vi "TDMSAdv readData.vi"(6 "stringSplit? (T)":bool=TRUE, 7 "readEvent":T1, 8 "error in (no error)":errorcluster, 10 "timeStamp":string, 11 "TDMSAdv in":refnum<class "TDMSAdv.lvclass">) -> (0 "error out":errorcluster, 2 "outputArr":string[][](array[string]), 3 "TDMSAdv out":refnum<class "TDMSAdv.lvclass">, 5 "getListTag":string[](array[string])=["TimeStamp", "SampleType", "mzRange"])   [LabVIEW 2018, in "TDMSAdv.lvclass"]
uses:
  TDMSAdv.lvclass
  FM/ctl/_PC_Pub_FM fileReadFuncEnum.ctl
  TDMSAdv.lvclass/TDMSAdv.ctl
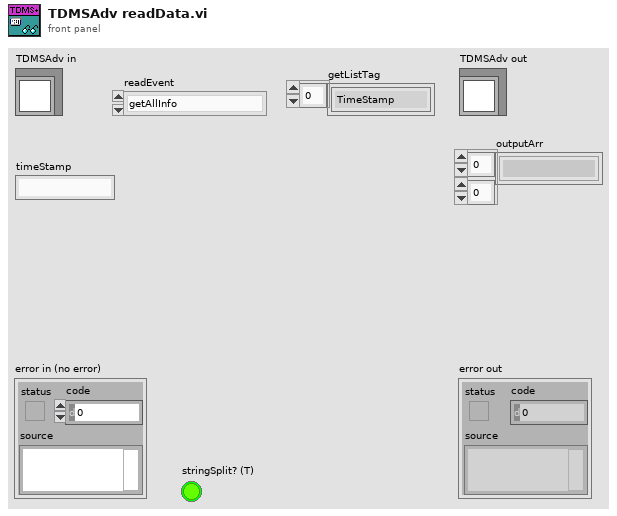
[diagram p1: front panel]
types:
  T1 = typedef "_PC_Pub_FM fileReadFuncEnum.ctl" = enum16{"getAllInfo", "getChromatogram", "getDataItems", "getTimeStamp", "getIdxData", "getIonization", "getRemark", "getAttrFormat"}
  T2 = enum16{"open", "open or create", "create or replace", "create", "open (read-only)"}
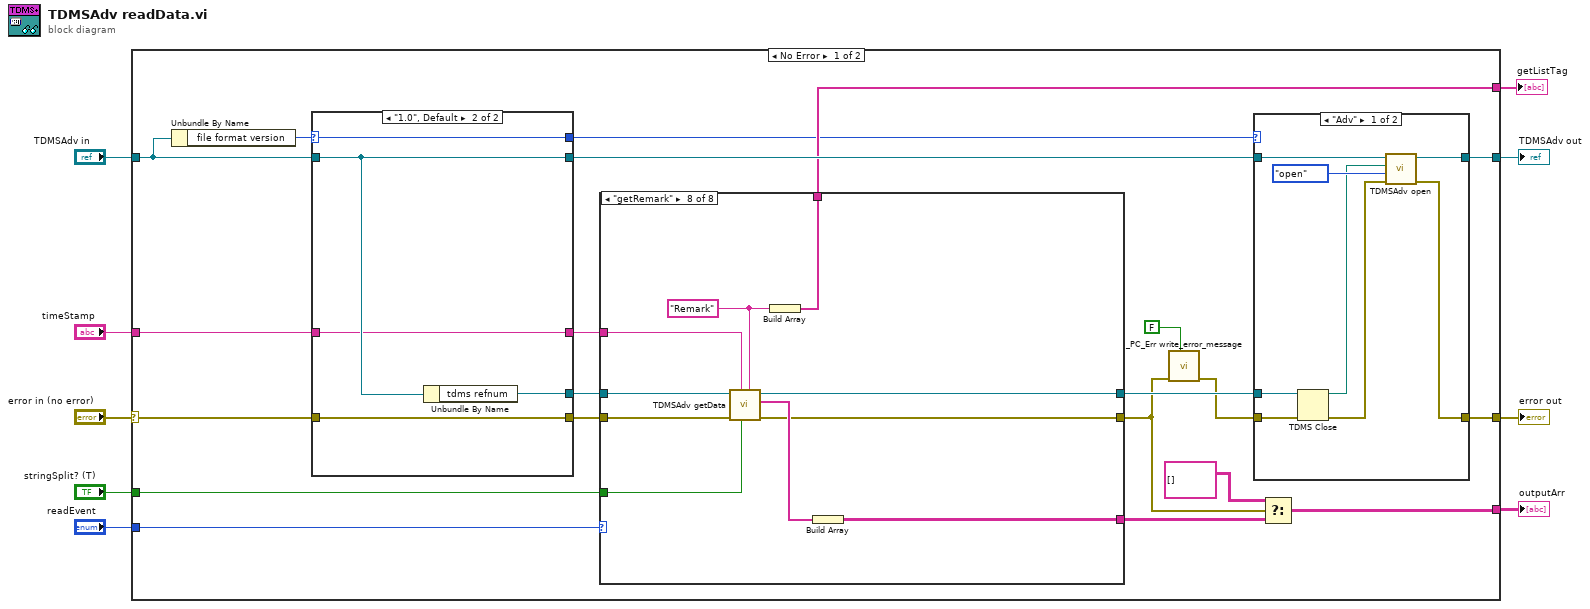
[diagram p0: block diagram]
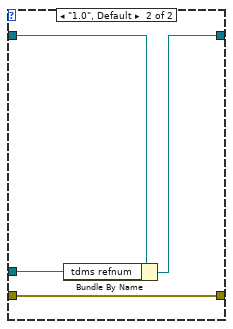
[diagram p2: hidden frame]
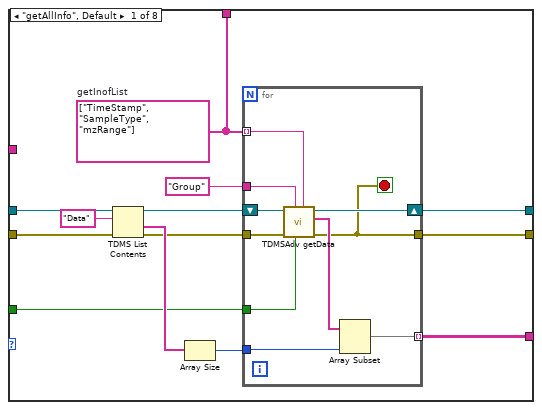
[diagram p3: hidden frame]
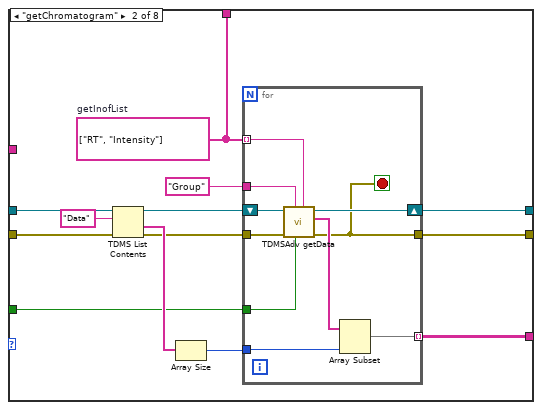
[diagram p4: hidden frame]
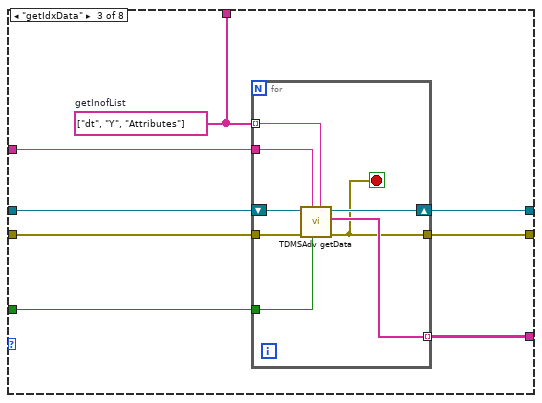
[diagram p5: hidden frame]
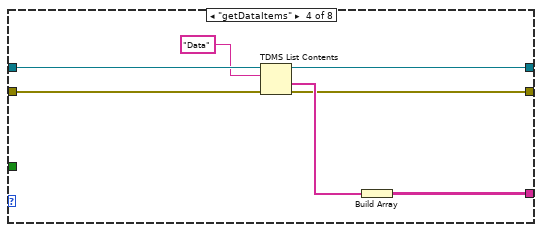
[diagram p6: hidden frame]
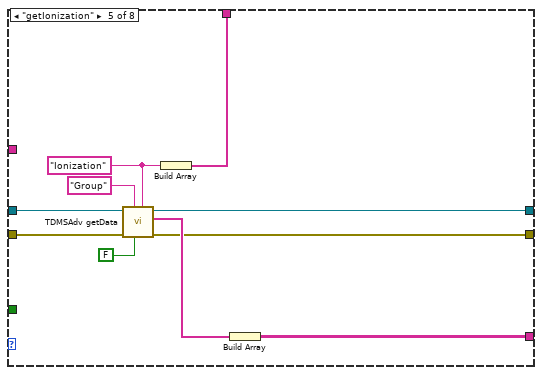
[diagram p7: hidden frame]
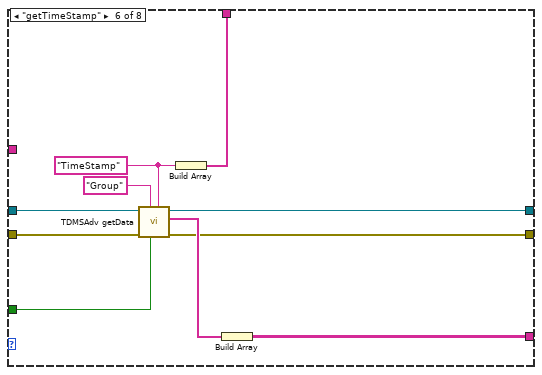
[diagram p8: hidden frame]
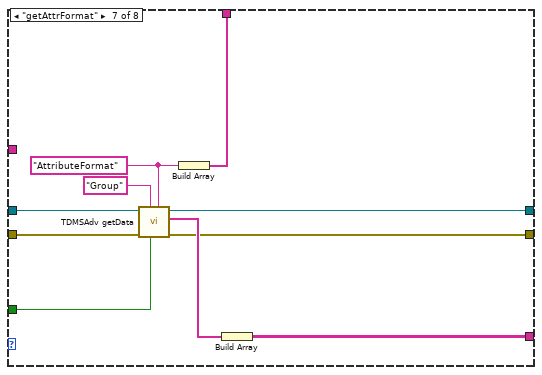
[diagram p9: hidden frame]
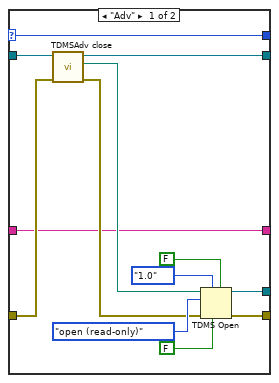
[diagram p10: hidden frame]
diagram:
  n1 = case shown="No Error" "error in (no error)" {
    selector: "error in (no error)" -> [w28 w170]
    tunnel: "TDMSAdv in" -> [w29 w171]
    tunnel: "timeStamp" -> [w20 _]
    tunnel: "readEvent" -> [w18 _]
    tunnel: "stringSplit? (T)" -> [w17 _]
    tunnel: [w15 _] -> w2
    tunnel: [w14 w170] -> w3
    tunnel: [w13 w171] -> w4
    tunnel: [w11 _] -> w1
    frame No Error {
      n2 = Unbundle By Name(w29) -> ("file format version"=w30:enum16{"1.0", "2.0", "Adv"})
      n3 = case shown="\"1.0\", Default" w30 {
        selector: w30 -> [w154 w166]
        tunnel: w29 -> [w164 w167]
        tunnel: [w157 w168] -> w27
        tunnel: [w156 w169] -> w26
        tunnel: w28 -> [w155 w169]
        tunnel: [w154 w166] -> w10
        tunnel: [w153 w167] -> w12
        tunnel: [w152 w165] -> w19
        tunnel: w20 -> [w152 w165]
        frame "Adv" {
          n4 = call "TDMSAdv close.vi"("error in (no error)"=w155, "TDMSAdv in"=w164) -> ("error out"=w158:errorcluster, "filePath"=w159:path, "TDMSAdv out"=w153:refnum<class "TDMSAdv.lvclass">)  [unwired: 7 in]
          n5 = TDMS Open(5:FALSE ("create index file? (T)"), 6:FALSE ("disable buffering (T)"), 7:enum16{"1.0", "2.0"}."1.0" ("file format version (2.0)"), 8:w158, 10:T2."open (read-only)" ("operation"), 11:w159) -> (0:w156:errorcluster, 3:w157:refnum<k34>)  [unwired: 1 in]
        }
        frame "1.0", Default {
          n6 = Unbundle By Name(w167) -> ("tdms refnum"=w168:refnum<k34>)
        }
      }
      n7 = case shown="\"getRemark\"" w18 {
        tunnel: w27 -> [w54 w77 w94 w111 w119 w129 w139 w150]
        tunnel: w26 -> [w53 w76 w93 w107 w115 w125 w135 w146]
        tunnel: [w45 w68 w92 w108 w117 w127 w137 w148] -> w21
        tunnel: [w47 w70 w96 w105 w118 w128 w138 w149] -> w24
        tunnel: [w46 w69 w95 w106 w116 w126 w136 w147] -> w22
        tunnel: w19 -> [_ _ w91 _ _ _ _ w142]
        tunnel: w17 -> [w43 w66 w89 _ _ w122 w132 w143]
        tunnel: [w44 w67 w90 _ w113 w123 w133 w144] -> w11
        frame "getAllInfo", Default {
          w44 = string[] ["TimeStamp", "SampleType", "mzRange"]  # getInofList
          n8 = TDMS List Contents(4:w53, 6:"Data" ("group name"), 7:w54) -> (0:w49:errorcluster, 1:w52:string[], 3:w50:refnum<k34>)  [unwired: 1 out]
          n9 = Array Size(array=w52) -> (size(s)=w51:i32)
          n10 = for {
            tunnel: w51 -> [w65]
            tunnel: w49 -> [w61]
            tunnel: w44 -> [w62] mode=indexing
            tunnel: "Group" ("group name") -> [w63]
            tunnel: [w64] -> w45 mode=indexing
            shift-right: [w58] -> w47
            shift-left: w50 -> [w60]
            tunnel: [w57] -> w46
            tunnel: w43 -> [w56]
            stop <- w57 stop-if-true
            n11 = call "TDMSAdv getData.vi"("channel name"=w62, "stringSplit? (T)"=w56, "group name"=w63, "error in (no error)"=w61, "tdms1.0 file"=w60) -> ("error out"=w57:errorcluster, "dataArr"=w59:string[], "tdms1.0 file out"=w58:refnum<k34>)  [unwired: 4 in]
            n12 = Array Subset(array=w59, length=w65) -> (w64:string[])  [unwired: 1 in]
          }
        }
        frame "getChromatogram" {
          w67 = string[] ["RT", "Intensity"]  # getInofList
          n13 = TDMS List Contents(4:w76, 6:"Data" ("group name"), 7:w77) -> (0:w72:errorcluster, 1:w75:string[], 3:w73:refnum<k34>)  [unwired: 1 out]
          n14 = Array Size(array=w75) -> (size(s)=w74:i32)
          n15 = for {
            tunnel: w74 -> [w88]
            tunnel: w72 -> [w84]
            tunnel: w67 -> [w85] mode=indexing
            tunnel: "Group" ("group name") -> [w86]
            tunnel: [w87] -> w68 mode=indexing
            shift-right: [w81] -> w70
            shift-left: w73 -> [w83]
            tunnel: [w80] -> w69
            tunnel: w66 -> [w79]
            stop <- w80 stop-if-true
            n16 = call "TDMSAdv getData.vi"("channel name"=w85, "stringSplit? (T)"=w79, "group name"=w86, "error in (no error)"=w84, "tdms1.0 file"=w83) -> ("error out"=w80:errorcluster, "dataArr"=w82:string[], "tdms1.0 file out"=w81:refnum<k34>)  [unwired: 4 in]
            n17 = Array Subset(array=w82, length=w88) -> (w87:string[])  [unwired: 1 in]
          }
        }
        frame "getIdxData" {
          w90 = string[] ["dt", "Y", "Attributes"]  # getInofList
          n18 = for {
            tunnel: w93 -> [w103]
            tunnel: w90 -> [w104] mode=indexing
            shift-right: [w101] -> w96
            shift-left: w94 -> [w102]
            tunnel: [w98] -> w95
            tunnel: w91 -> [w100]
            tunnel: [w99] -> w92 mode=indexing
            tunnel: w89 -> [w97]
            stop <- w98 stop-if-true
            n19 = call "TDMSAdv getData.vi"("channel name"=w104, "stringSplit? (T)"=w97, "group name"=w100, "error in (no error)"=w103, "tdms1.0 file"=w102) -> ("error out"=w98:errorcluster, "dataArr"=w99:string[], "tdms1.0 file out"=w101:refnum<k34>)  [unwired: 4 in]
          }
        }
        frame "getDataItems" {
          n20 = TDMS List Contents(4:w107, 6:"Data" ("group name"), 7:w111) -> (0:w106:errorcluster, 1:w109:string[], 3:w105:refnum<k34>)  [unwired: 1 out]
          n21 = Build Array(w109) -> (w108:string[][])
        }
        frame "getIonization" {
          w114 = "Ionization" ("group name")
          n22 = call "TDMSAdv getData.vi"("channel name"=w114, "stringSplit? (T)"=FALSE, "group name"="Group", "error in (no error)"=w115, "tdms1.0 file"=w119) -> ("error out"=w116:errorcluster, "dataArr"=w120:string[], "tdms1.0 file out"=w118:refnum<k34>)  [unwired: 4 in]
          n23 = Build Array(w114) -> (w113:string[])
          n24 = Build Array(w120) -> (w117:string[][])
        }
        frame "getTimeStamp" {
          w124 = "TimeStamp" ("group name")
          n25 = call "TDMSAdv getData.vi"("channel name"=w124, "stringSplit? (T)"=w122, "group name"="Group", "error in (no error)"=w125, "tdms1.0 file"=w129) -> ("error out"=w126:errorcluster, "dataArr"=w130:string[], "tdms1.0 file out"=w128:refnum<k34>)  [unwired: 4 in]
          n26 = Build Array(w124) -> (w123:string[])
          n27 = Build Array(w130) -> (w127:string[][])
        }
        frame "getAttrFormat" {
          w134 = "AttributeFormat" ("group name")
          n28 = call "TDMSAdv getData.vi"("channel name"=w134, "stringSplit? (T)"=w132, "group name"="Group", "error in (no error)"=w135, "tdms1.0 file"=w139) -> ("error out"=w136:errorcluster, "dataArr"=w140:string[], "tdms1.0 file out"=w138:refnum<k34>)  [unwired: 4 in]
          n29 = Build Array(w134) -> (w133:string[])
          n30 = Build Array(w140) -> (w137:string[][])
        }
        frame "getRemark" {
          w145 = "Remark" ("group name")
          n31 = call "TDMSAdv getData.vi"("channel name"=w145, "stringSplit? (T)"=w143, "group name"=w142, "error in (no error)"=w146, "tdms1.0 file"=w150) -> ("error out"=w147:errorcluster, "dataArr"=w151:string[], "tdms1.0 file out"=w149:refnum<k34>)  [unwired: 4 in]
          n32 = Build Array(w145) -> (w144:string[])
          n33 = Build Array(w151) -> (w148:string[][])
        }
      }
      n34 = call "_PC_Err write_error_message.vi"("show msg( T )"=FALSE, "error in"=w22) -> ("error out"=w23:errorcluster)  [unwired: 9 in]
      n35 = case shown="\"Adv\"" w10 {
        tunnel: w12 -> [w35 w41]
        tunnel: [w32 w42] -> w14
        tunnel: w23 -> [w37 w42]
        tunnel: w24 -> [w38 w40]
        tunnel: [w31 w39] -> w13
        frame "Adv" {
          n36 = TDMS Close(8:w37, 11:w38) -> (0:w33:errorcluster, 3:w34:path)
          n37 = call "TDMSAdv open.vi"("error in (no error)"=w33, "operation (0:open)"=T2."open", "openPath"=w34, "TDMSAdv in"=w35) -> ("error out"=w32:errorcluster, "TDMSAdv out"=w31:refnum<class "TDMSAdv.lvclass">)  [unwired: 6 in]
        }
        frame "1.0", Default {
          n38 = Bundle By Name(cluster=w41, "tdms refnum"=w40) -> (w39:refnum<class "TDMSAdv.lvclass">)
        }
      }
      n39 = Select(t=string[][] [], s=w22, f=w21) -> (s? t:f=w15:string[][])
    }
    frame Error {
    }
  }
  "error out" <- w3
  "TDMSAdv out" <- w4
  "outputArr" <- w2
  "getListTag" <- w1
